vi "getData_v11.vi"() -> ()   [LabVIEW 2014]
uses:
  <vilib>/rvi/interface/nirviOpenFPGA/nirviOpenFPGA.xnode
  <vilib>/rvi/interface/nirviCloseFPGA/nirviCloseFPGA.xnode
  <vilib>/FPGAPlugInAG/Dynamic/niLvFpga_Close_Dynamic.vi
  <vilib>/Utility/file.llb/Write To Spreadsheet File (DBL).vi
  <vilib>/rvi/interface/nirviReadWriteControl/nirviReadWriteControl.xnode
  <vilib>/rvi/interface/Simulation/niFpgaSimulationCallBeginRW.vi
  <vilib>/rvi/errors/niLvFpgaAdjustHostInterfaceError.vi
panel:
  out "message":string=" INSTRUCTIONS:\r\rNormal Use:  When using subVIs that incorporate the error in/error out (or error I/O) structure, place this handler where you want to inform the user of an error, typically at the end of the I/O data path, as the last action of the program.  If the error in error? is ERROR, the handler creates a message describing the error and its source.  If the type of dialog = 1 (default), the message is displayed to the user, who can only acknowedge it.  If the type = 2, the user can acknowledge the message or abort execution; aborting a program with active I/O is not recommended.  If the type = 0, no message is displayed; this is used to process the error programmatically, and the error out cluster elements are wired to individual terminals for that reason.  \r\rOther Use:\n\r\nlocal testing.  To test the error code of a subVI or function that does not have the error I/O structure, you can wire its error code and a source string to the local error code and error source inputs.  If error in error? indicates no error and error code is not equal to 0, the local code and source are substituted for the error in values, and error? is set TRUE (ERROR)."
  out "time out?":bool
  in  "Time Read":i32
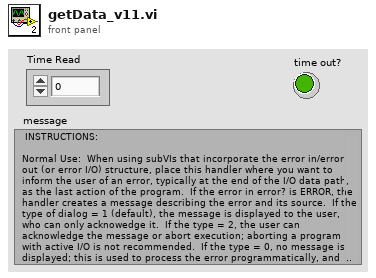
[diagram p1: front panel]
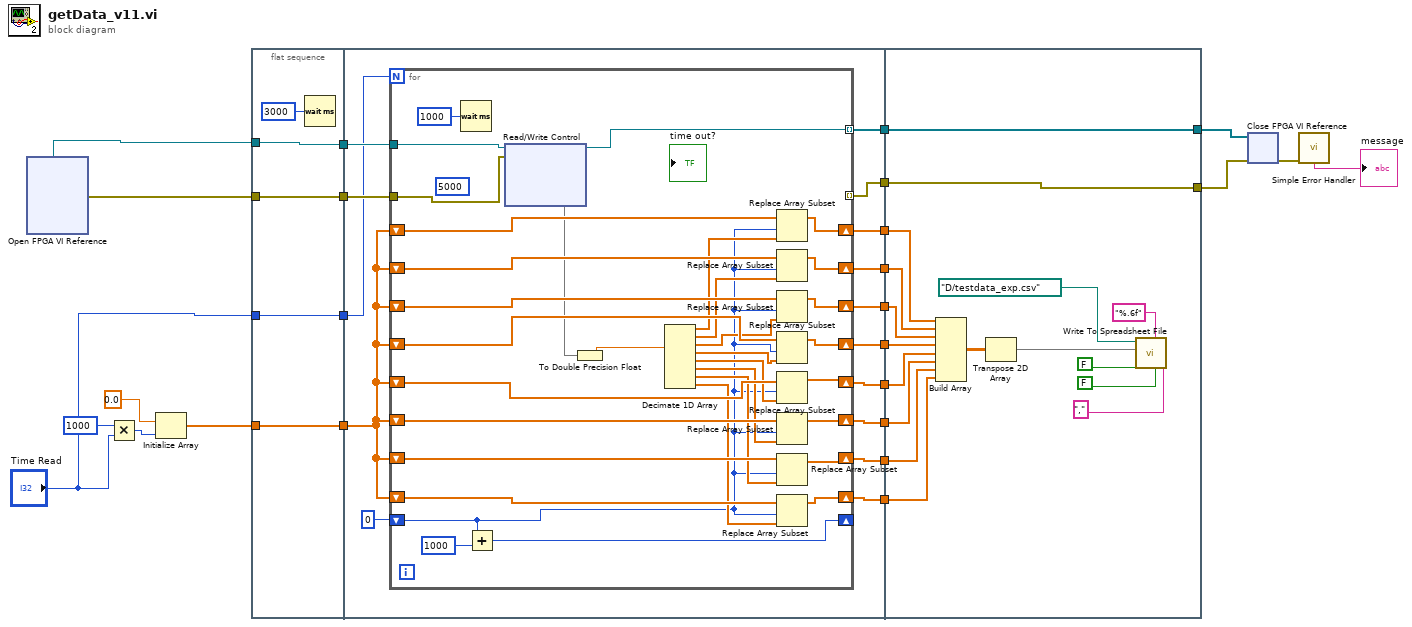
[diagram p0: block diagram]
diagram:
  n1 = xnode "Open FPGA VI Reference"() -> ("FPGA VI Reference Out"=w22:refnum<k20>, "error out"=w20:errorcluster)  [unwired: 2 in]
  n2 = Multiply(x=1000, y="Time Read") -> (x*y=w16:i32)
  n3 = Initialize Array(0.0 ("element"), w16) -> (w12:dbl[])
  n4 = flat-sequence {
    tunnel: w22 -> [w29]
    tunnel: [w29] -> w21
    tunnel: w20 -> [w28]
    tunnel: [w28] -> w19
    tunnel: "Time Read" -> [w27]
    tunnel: [w27] -> w13
    tunnel: w12 -> [w26]
    tunnel: [w26] -> w11
    tunnel: [w43] -> w23
    tunnel: w21 -> [w45]
    tunnel: w19 -> [w44]
    tunnel: [w42] -> w18
    tunnel: w13 -> [w41]
    tunnel: w11 -> [w39]
    tunnel: [w38] -> w10
    tunnel: [w37] -> w9
    tunnel: [w36] -> w8
    tunnel: [w35] -> w7
    tunnel: [w34] -> w6
    tunnel: [w33] -> w5
    tunnel: [w32] -> w4
    tunnel: [w31] -> w3
    tunnel: [w96] -> w2
    tunnel: w23 -> [w96]
    tunnel: w18 -> [w95]
    tunnel: [w95] -> w1
    tunnel: w10 -> [w94]
    tunnel: w9 -> [w93]
    tunnel: w8 -> [w92]
    tunnel: w7 -> [w91]
    tunnel: w6 -> [w90]
    tunnel: w5 -> [w89]
    tunnel: w4 -> [w88]
    tunnel: w3 -> [w87]
    frame #0 {
      n5 = Wait (ms)(milliseconds to wait=u32 3000) -> ()  [unwired: 1 out]
    }
    frame #1 {
      n6 = for {
        N: w41 -> [_]
        tunnel: [_] -> w43 mode=indexing
        tunnel: w45 -> [w48]
        tunnel: w44 -> [w47]
        tunnel: [w50] -> w42 mode=indexing
        shift-right: [w69] -> w38
        shift-left: w39 -> [w77]
        shift-right: [w68] -> w37
        shift-left: w39 -> [w76]
        shift-right: [w67] -> w36
        shift-left: w39 -> [w75]
        shift-right: [w66] -> w35
        shift-left: w39 -> [w74]
        shift-right: [w65] -> w34
        shift-left: w39 -> [w73]
        shift-right: [w64] -> w33
        shift-left: w39 -> [w72]
        shift-right: [w63] -> w32
        shift-left: w39 -> [w71]
        shift-right: [w62] -> w31
        shift-left: w39 -> [w70]
        shift-right: [w78] -> _
        shift-left: 0 -> [w53]
        (unwired) 5000 ("timeout in ms (0)")
        n7 = Wait (ms)(milliseconds to wait=u32 1000) -> ()  [unwired: 1 out]
        n8 = Add(x=w53, y=1000) -> (x+y=w78:i32)
        n9 = xnode "Read/Write Control"("FPGA VI Reference In"=w48, "error in"=w47) -> ("FPGA VI Reference Out"=w50:refnum<k20>, "error out"=w49:errorcluster, "Unselected"=w46)  [unwired: 2 in]
        n10 = To Double Precision Float(number=w46) -> (double precision float=w51:dbl)
        n11 = Decimate 1D Array(w51) -> (w54:dbl[], w55:dbl[], w56:dbl[], w57:dbl[], w58:dbl[], w59:dbl[], w60:dbl[], w61:dbl[])
        n12 = Replace Array Subset(array=w77, new element=w54, index=w53) -> (w69:dbl[])
        n13 = Replace Array Subset(array=w76, new element=w55, index=w53) -> (w68:dbl[])
        n14 = Replace Array Subset(array=w75, new element=w56, index=w53) -> (w67:dbl[])
        n15 = Replace Array Subset(array=w74, new element=w57, index=w53) -> (w66:dbl[])
        n16 = Replace Array Subset(array=w73, new element=w58, index=w53) -> (w65:dbl[])
        n17 = Replace Array Subset(array=w72, new element=w59, index=w53) -> (w64:dbl[])
        n18 = Replace Array Subset(array=w71, new element=w60, index=w53) -> (w63:dbl[])
        n19 = Replace Array Subset(array=w70, new element=w61, index=w53) -> (w62:dbl[])
      }
    }
    frame #2 {
      n20 = Build Array(w94, w93, w92, w91, w90, w89, w88, w87) -> (w86:dbl[][])
      n21 = Transpose 2D Array(2D array=w86) -> (transposed array=w84:dbl[][])
      n22 = call-poly <vilib>:"Write To Spreadsheet File.vi"("delimiter (\\t)"=",", "transpose? (no:F)"=FALSE, "format (%.3f)"="%.6f", "append to file? (new file:F)"=FALSE, "2D data"=w84, "file path (dialog if empty)"=path "D:/testdata_exp.csv") -> ()  [unwired: 2 in, 1 out]
    }
  }
  n23 = xnode "Close FPGA VI Reference"("FPGA VI Reference In"=w1, "error in"=w2) -> ("error out"=w24:errorcluster)
  n24 = call <vilib>:"Simple Error Handler.vi"("error in (no error)"=w24) -> ("message"=→"message":string)  [unwired: 4 in, 4 out]
